vi "DeviceRead.vi"(4 "error in (no error)":errorcluster, 7 "CmdLib In":refnum<k24>) -> (0 "error out":errorcluster, 1 "Response":string, 3 "CmdLib Out":refnum<k24>)   [LabVIEW 2013]
uses:
  C:/Code/Apps/Utilities/AG-UC2-UC8/AG-UC2-UC8/Install/Samples/LabVIEW/LabVIEW 2013/CmdLibAgilis.dll
  CmdLibAgilis.dll
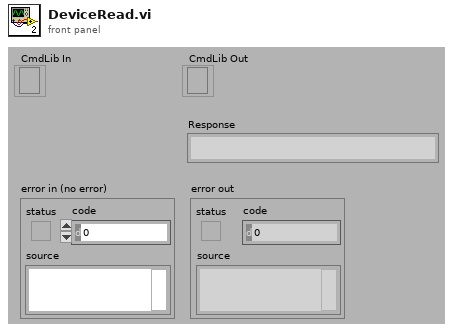
[diagram p1: front panel]
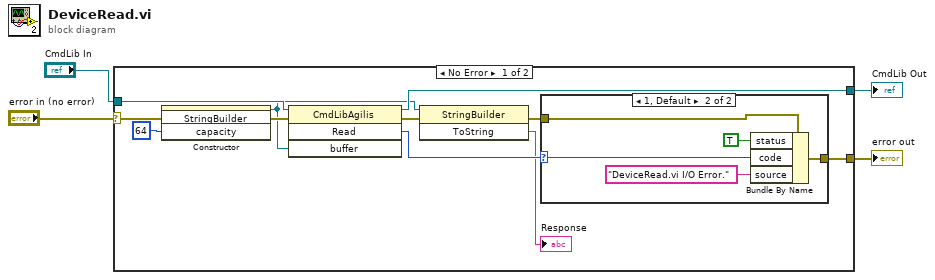
[diagram p0: block diagram]
diagram:
  n1 = case shown="No Error" "error in (no error)" {
    selector: "error in (no error)" -> [w12 w23]
    tunnel: [w7 w23] -> w3
    tunnel: "CmdLib In" -> [w15 w22]
    tunnel: [w14 w22] -> w1
    frame No Error {
      n2 = constructor class="StringBuilder"(error in=w12, "capacity"=64) -> (reference out=w5:refnum<k24>, error out=w11:errorcluster)  [unwired: 2 in, 2 out]
      n3 = invoke class="CmdLibAgilis" method="Read"(reference=w15, error in=w11, "buffer"=w5) -> (reference out=w14:refnum<k24>, error out=w10:errorcluster, "Read"=w9:i32)  [unwired: 1 in, 1 out]
      n4 = invoke class="StringBuilder" method="ToString"(reference=w5, error in=w10) -> (error out=w8:errorcluster, "ToString"=→"Response":string)  [unwired: 1 in, 1 out]
      n5 = case shown="1, Default" w9 {
        selector: w9 -> [_ w17]
        tunnel: w8 -> [w16 w19]
        tunnel: [w16 w18] -> w7
        frame 0 {
        }
        frame 1, Default {
          n6 = Bundle By Name(cluster=w19, "status"=TRUE, "code"=w17, "source"="DeviceRead.vi I/O Error.") -> (w18:errorcluster)
        }
      }
    }
    frame Error {
    }
  }
  "error out" <- w3
  "CmdLib Out" <- w1
